vi "9.-Uso de Gráfica XY.vi"() -> ()   [LabVIEW 2020]
panel:
  in  "stop":bool
  out "XY Graph 2":cluster{"Y":dbl[], "Y":dbl[]}[](graph)
  out "XY Graph":cluster{dbl[], dbl[]}(graph)
  in  "Knob":i32(knob)=100 scale=0.0..1000.0
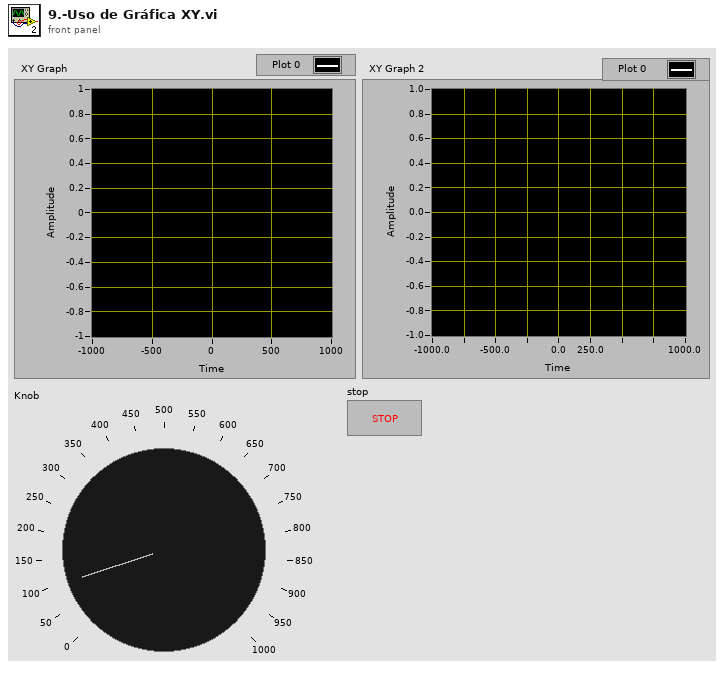
[diagram p1: front panel]
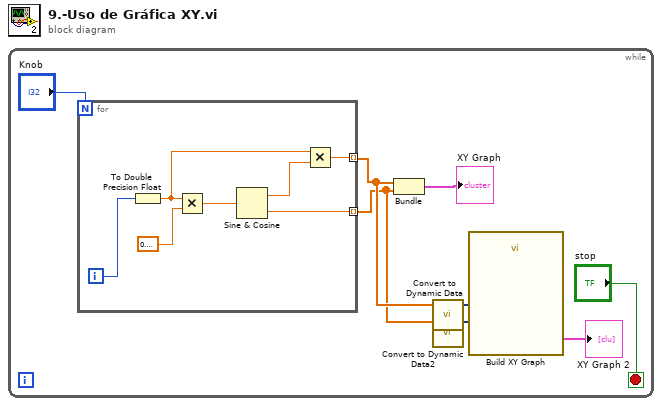
[diagram p0: block diagram]
diagram:
  n1 = while {
    stop <- "stop" stop-if-true
    n2 = for {
      N: "Knob" -> [_]
      tunnel: [w10] -> w5 mode=indexing
      tunnel: [w9] -> w3 mode=indexing
      i -> [w15]
      n3 = To Double Precision Float(number=w15) -> (double precision float=w11:dbl)
      n4 = Multiply(x=w11, y=0.3183098861837907) -> (x*y=w13:dbl)
      n5 = Sine & Cosine(0:w13) -> (1:w12:dbl, 2:w9:dbl)
      n6 = Multiply(x=w11, y=w12) -> (x*y=w10:dbl)
    }
    n7 = Bundle(w5, w3) -> (→"XY Graph":cluster{dbl[], dbl[]})  [unwired: 1 in]
    n8 = call "Convert to Dynamic Data"("Array"=w5) -> ("Dynamic Data Type"=w4:dynamicdata)  [unwired: 3 in]
    n9 = call "Convert to Dynamic Data2"("Array"=w3) -> ("Dynamic Data Type"=w2:dynamicdata)  [unwired: 3 in]
    n10 = call "Build XY Graph"("Y Input"=w2, "X Input"=w4) -> ("XY Graph"=→"XY Graph 2":cluster{"X":dbl[], "Y":dbl[]}[])  [unwired: 8 in, 1 out]
  }
